vi "Start.vi"(8 "error in (no error)":errorcluster, 10 "Message in":refnum<class "StartMessage.lvclass">, 11 "DAQMH121119OrcaFlash in":refnum<class "DAQOrcaFlash.lvclass">) -> (0 "error out":errorcluster, 3 "DAQMH121119OrcaFlash out":refnum<class "DAQOrcaFlash.lvclass">)   [LabVIEW 2012, in "DAQOrcaFlash.lvclass"]
doc: "This member function is called when the statemachine in the run.vi receives an 'start' command. It relays the message to all observers of the component.\n\nOverride this member function in your derived class if you need additional start functionality (but don't forget to call the parent method)."
uses:
  DAQOrcaFlash.lvclass
  <vilib>/Distrio/Murmex/StartMessage/StartMessage.lvclass
  <vilib>/Distrio/Murmex/Murmex/Murmex.lvclass
  DAQOrcaFlash.lvclass/DAQOrcaFlash.ctl
  imaging_mode.ctl
  trigger_source.ctl
  trigger_mode.ctl
  <vilib>/Distrio/Murmex/ResetMessage/ResetMessage.lvclass
  <vilib>/Distrio/Murmex/Message/Message.lvclass
panel:
  # "This method is called when the START\ntrigger is sent. \n\nOverride this method when your component needs to\nrespond to this trigger. \n\nCall parent for proper implementation"
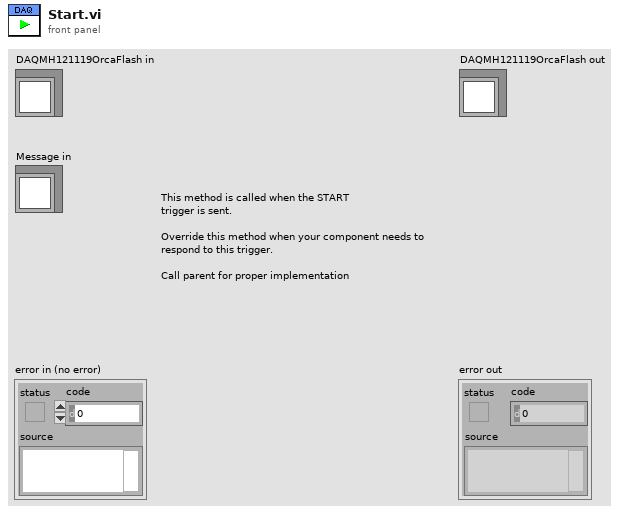
[diagram p1: front panel]
types:
  T1 = typedef "DAQOrcaFlash.lvclass/imaging_mode.ctl" = enum16{"focus mode", "single sweep"}
  T2 = typedef "Murmex.lvlib/StartMessage.lvclass/run mode enum.ctl" = enum16{"infinite", "finite"}
  T3 = typedef "DAQOrcaFlash.lvclass/trigger_mode.ctl" = sgl
  T4 = typedef "DAQOrcaFlash.lvclass/trigger_source.ctl" = sgl
  T5 = typedef "IMAQ Image.ctl" = refnum<image>
  T6 = cluster{"height":u32, "width":u32, "datatype":u32}
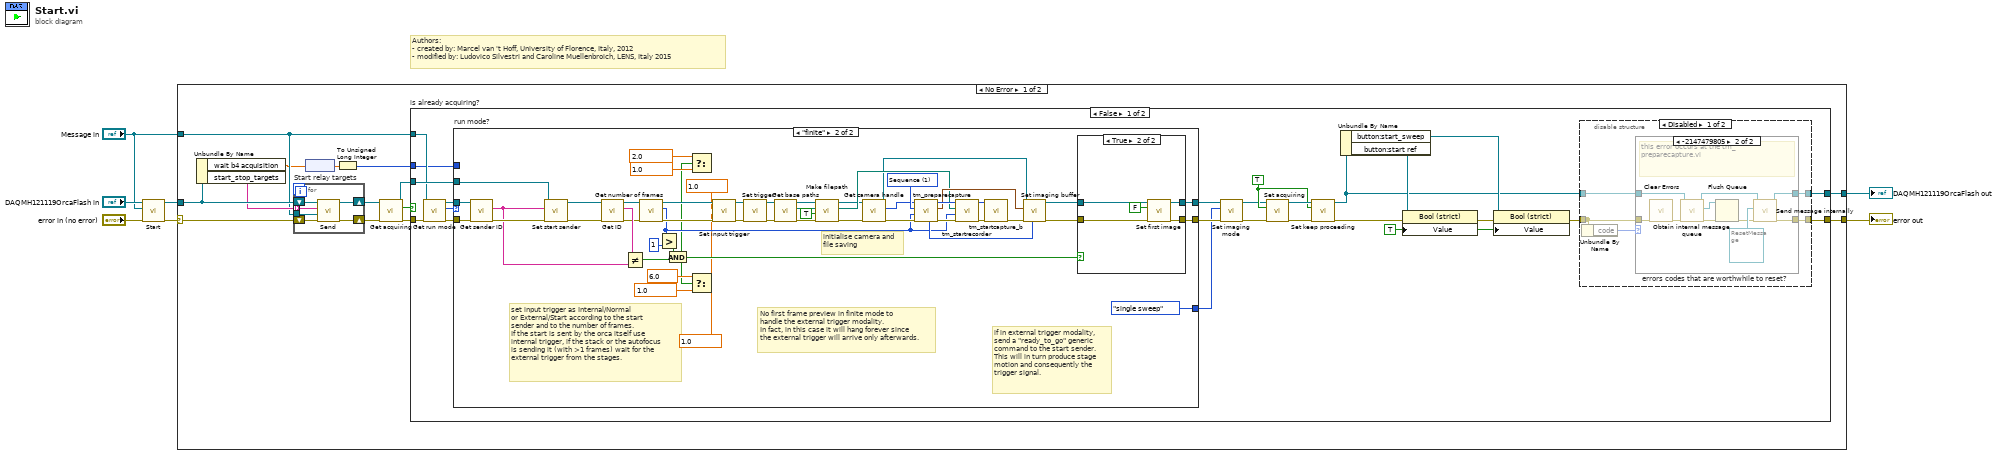
[diagram p0: block diagram]
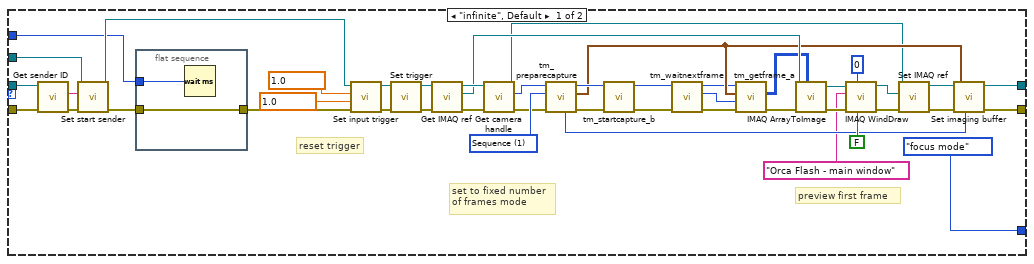
[diagram p4: hidden frame]
diagram:
  # "Authors: \n- created by: Marcel van 't Hoff, University of Florence, Italy, 2012\n- modified by: Ludovico Silvestri and Caroline Muellenbroich, LENS, Italy 2015"
  n1 = call-parent "Start.vi"("error in (no error)"="error in (no error)", "Message in"="Message in", "Murmex in"="DAQMH121119OrcaFlash in") -> ("error out"=w3:errorcluster, "Murmex out"=w4:refnum<class "DAQOrcaFlash.lvclass">)  [unwired: 7 in]
  n2 = case shown="No Error" w3 {
    selector: w3 -> [w14 w178]
    tunnel: [w21 w178] -> w2
    tunnel: [w20 w177] -> w7
    tunnel: w4 -> [w16 w177]
    tunnel: "Message in" -> [w13 _]
    frame No Error {
      n3 = Unbundle By Name(w16) -> ("wait b4 acquisition"=w12:dbl[unit], "start_stop_targets"=w15:string[])
      n4 = for "Start relay targets" {
        shift-right: [w27] -> w9
        shift-left: w14 -> [w26]
        tunnel: w13 -> [w24]
        tunnel: w15 -> [w23] mode=indexing
        shift-right: [w22] -> w10
        shift-left: w16 -> [w25]
        n5 = call <vilib>:"Send.vi"("error in (no error)"=w26, "Message"=w24, "recipient"=w23, "Murmex in"=w25) -> ("error out"=w27:errorcluster, "Murmex out"=w22:refnum<class "DAQOrcaFlash.lvclass">)  [unwired: 6 in]
      }
      n6 = node(w12) -> (w11:dbl)
      n7 = To Unsigned Long Integer(number=w11) -> (unsigned 32bit integer=w8:u32)
      n8 = call "Get acquiring.vi"("error in (no error)"=w9, "DAQMH121119OrcaFlash in"=w10) -> ("error out"=w18:errorcluster, "is acquiring?"=w17:bool, "DAQMH121119OrcaFlash out"=w19:refnum<class "DAQOrcaFlash.lvclass">)  [unwired: 7 in]
      n9 = case "is already acquiring?" shown="False" w17 {
        tunnel: [w38 w176] -> w21
        tunnel: [w36 w175] -> w20
        tunnel: w19 -> [w46 w175]
        tunnel: w18 -> [w42 w176]
        tunnel: w13 -> [w39 _]
        tunnel: w8 -> [w32 _]
        frame False {
          w49 = TRUE ("Value")
          w33 = TRUE ("is acquiring?")
          n10 = call <vilib>:"Get run mode.vi"("error in (no error)"=w42, "StartMessage in"=w39) -> ("error out"=w41:errorcluster, "run mode"=w40:T2, "StartMessage out"=w35:refnum<class "StartMessage.lvclass">)  [unwired: 7 in]
          n11 = case "run mode?" shown="\"finite\"" w40 {
            tunnel: w41 -> [w77 w152]
            tunnel: [w112 w128] -> w51
            tunnel: [w113 w126] -> w45
            tunnel: w46 -> [w75 w124]
            tunnel: [imaging_mode."focus mode" ("imaging mode") imaging_mode."single sweep" ("imaging mode")] -> w44
            tunnel: w35 -> [w76 w151]
            tunnel: w32 -> [w71 _]
            frame "infinite", Default {
              w80 = T3 1.0 items=["Normal"=1.0, "Start"=6.0] ("Trigger mode")
              w81 = T4 1.0 items=["Internal"=1.0, "External"=2.0, "Software"=3.0] ("Trigger source")
              w105 = 1 items=["Snap", "Sequence"] ("Capture mode")
              # "reset trigger"
              # "preview first frame"
              # "set to fixed number\nof frames mode"
              n12 = call <vilib>:"Get sender ID.vi"("error in (no error)"=w77, "Message in"=w76) -> ("error out"=w79:errorcluster, "sender"=w78:string)  [unwired: 7 in, 1 out]
              n13 = call-dynamic "Set start sender.vi"("error in (no error)"=w79, "start sender"=w78, "DAQOrcaFlash in"=w75) -> ("error out"=w72:errorcluster, "DAQOrcaFlash out"=w74:refnum<class "DAQOrcaFlash.lvclass">)  [unwired: 7 in]
              n14 = flat-sequence {
                tunnel: [w117] -> w73
                tunnel: w72 -> [w117]
                tunnel: w71 -> [w116]
                frame #0 {
                  n15 = Wait (ms)(milliseconds to wait=w116) -> ()  [unwired: 1 out]
                }
              }
              n16 = call-dynamic "Set input trigger.vi"("error in (no error)"=w73, "Trigger mode"=w80, "Trigger source"=w81, "DAQOrcaFlash in"=w74) -> ("error out"=w83:errorcluster, "DAQOrcaFlash out"=w84:refnum<class "DAQOrcaFlash.lvclass">)  [unwired: 6 in]
              n17 = call-dynamic "Set trigger.vi"("error in (no error)"=w83, "DAQOrcaFlash in"=w84) -> ("error out"=w82:errorcluster, "DAQOrcaFlash out"=w85:refnum<class "DAQOrcaFlash.lvclass">)  [unwired: 8 in]
              n18 = call "Get IMAQ ref.vi"("error in (no error)"=w82, "DAQMH121119OrcaFlash in"=w85) -> ("error out"=w114:errorcluster, "IMAQ reference"=w99:T5, "DAQMH121119OrcaFlash out"=w115:refnum<class "DAQOrcaFlash.lvclass">)  [unwired: 7 in]
              n19 = call "Get camera handle.vi"("error in (no error)"=w114, "DAQMH121119OrcaFlash in"=w115) -> ("error out"=w88:errorcluster, "cam handle"=w89:u32, "DAQMH121119OrcaFlash out"=w92:refnum<class "DAQOrcaFlash.lvclass">)  [unwired: 7 in]
              n20 = call <userlib>:"tm_preparecapture.vi"("error in (no error)"=w88, "Capture mode"=w105, "Handle in"=w89) -> ("error out"=w106:errorcluster, "Buffer Info"=w97:T6, "Handle out"=w104:u32, "Image type"=w96:u32)  [unwired: 5 in]
              n21 = call <userlib>:"tm_startcapture_b.vi"("error in (no error)"=w106, "Handle in"=w104) -> ("error out"=w102:errorcluster, "Handle out"=w103:u32)  [unwired: 8 in]
              n22 = call <userlib>:"tm_waitnextframe.vi"("error in (no error)"=w102, "Handle in"=w103) -> ("error out"=w87:errorcluster, "Frame Index"=w101:i32, "Handle out"=w86:u32)  [unwired: 6 in, 1 out]
              n23 = call <userlib>:"tm_getframe_a.vi"("error in (no error)"=w87, "Frame Index"=w101, "Buffer Info"=w97, "Handle in"=w86) -> ("error out"=w93:errorcluster, "Data 16"=w95:u16[][])  [unwired: 3 in, 3 out]
              n24 = call "IMAQ ArrayToImage"("Image Pixels (U16)"=w95, "error in (no error)"=w93, "Image"=w99) -> ("error out"=w100:errorcluster, "Image Out"=w98:T5)  [unwired: 7 in]
              n25 = call "IMAQ WindDraw"("Resize to Image Size? (Y)"=FALSE, "Window Number (0...15)"=0, "error in (no error)"=w100, "Title"="Orca Flash - main window", "Image"=w98) -> ("error out"=w108:errorcluster, "Image Out (duplicate)"=w94:T5)  [unwired: 5 in]
              n26 = call "Set IMAQ ref.vi"("error in (no error)"=w108, "IMAQ reference"=w94, "DAQMH121119OrcaFlash in"=w92) -> ("error out"=w109:errorcluster, "DAQMH121119OrcaFlash out"=w110:refnum<class "DAQOrcaFlash.lvclass">)  [unwired: 7 in]
              n27 = call "Set imaging buffer.vi"("Image type"=w96, "error in (no error)"=w109, "Buffer"=w97, "DAQMH121119OrcaFlash in"=w110) -> ("error out"=w112:errorcluster, "DAQMH121119OrcaFlash out"=w113:refnum<class "DAQOrcaFlash.lvclass">)  [unwired: 6 in]
            }
            frame "finite" {
              w118 = T3 1.0 items=["Normal"=1.0, "Start"=6.0] ("Trigger mode")
              w119 = T4 1.0 items=["Internal"=1.0, "External"=2.0, "Software"=3.0] ("Trigger source")
              w142 = T3 1.0 items=["Normal"=1.0, "Start"=6.0] ("Trigger mode")
              w143 = T3 6.0 items=["Normal"=1.0, "Start"=6.0] ("Trigger mode")
              w145 = T4 1.0 items=["Internal"=1.0, "External"=2.0, "Software"=3.0] ("Trigger source")
              w144 = T4 2.0 items=["Internal"=1.0, "External"=2.0, "Software"=3.0] ("Trigger source")
              w165 = 1 items=["Snap", "Sequence"] ("Capture mode")
              # "if in external trigger modality,\nsend a \"ready_to_go\" generic\ncommand to the start sender.\nThis will in turn produce stage\nmotion and consequently the\ntrigger signal."
              # "No first frame preview in finite mode to\nhandle the external trigger modality.\nIn fact, in this case it will hang forever since\nthe external trigger will arrive only afterwards."
              # "set input trigger as Internal/Normal\nor External/Start according to the start\nsender and to the number of frames.\nIf the start is sent by the orca itself use\ninternal trigger, if the stack or the autofocus\nis sending it (with >1 frames) wait for the \nexternal trigger from the stages."
              # "initialise camera and\nfile saving"
              n28 = call <vilib>:"Get sender ID.vi"("error in (no error)"=w152, "Message in"=w151) -> ("error out"=w122:errorcluster, "sender"=w120:string)  [unwired: 7 in, 1 out]
              n29 = call-dynamic "Set start sender.vi"("error in (no error)"=w122, "start sender"=w120, "DAQOrcaFlash in"=w124) -> ("error out"=w121:errorcluster, "DAQOrcaFlash out"=w123:refnum<class "DAQOrcaFlash.lvclass">)  [unwired: 7 in]
              n30 = call <vilib>:"Get ID.vi"("error in (no error)"=w121, "Murmex in"=w123) -> ("error out"=w139:errorcluster, "component id"=w150:string, "Murmex out"=w141:refnum<class "DAQOrcaFlash.lvclass">)  [unwired: 7 in]
              n31 = Not Equal?(x=w150, y=w120) -> (x != y?=w133:bool)
              n32 = call "Get number of frames.vi"("error in (no error)"=w139, "DAQMH121119OrcaFlash in"=w141) -> ("error out"=w138:errorcluster, "no. of frames"=w135:i32, "DAQMH121119OrcaFlash out"=w140:refnum<class "DAQOrcaFlash.lvclass">)  [unwired: 7 in]
              n33 = Greater?(x=w135, y=1) -> (0:w132:bool)
              n34 = And(x=w132, y=w133) -> (x .and. y?=w125:bool)
              n35 = Select(t=w144, s=w125, f=w145) -> ()  [unwired: 1 out]
              n36 = Select(t=w143, s=w125, f=w142) -> ()  [unwired: 1 out]
              n37 = call-dynamic "Set input trigger.vi"("error in (no error)"=w138, "Trigger mode"=w118, "Trigger source"=w119, "DAQOrcaFlash in"=w140) -> ("error out"=w146:errorcluster, "DAQOrcaFlash out"=w147:refnum<class "DAQOrcaFlash.lvclass">)  [unwired: 6 in]
              n38 = call-dynamic "Set trigger.vi"("error in (no error)"=w146, "DAQOrcaFlash in"=w147) -> ("error out"=w149:errorcluster, "DAQOrcaFlash out"=w148:refnum<class "DAQOrcaFlash.lvclass">)  [unwired: 8 in]
              n39 = call-dynamic "Get base paths.vi"("error in (no error)"=w149, "DAQOrcaFlash in"=w148) -> ("error out"=w161:errorcluster, "filepath"=w159:path, "DAQOrcaFlash out"=w160:refnum<class "DAQOrcaFlash.lvclass">)  [unwired: 6 in, 1 out]
              n40 = call "Make filepath.vi"("error in (no error)"=w161, "is cxd file path?"=TRUE, "base path"=w159, "DAQOrcaFlash in"=w160) -> ("error out"=w136:errorcluster, "filepath out"=w158:path, "DAQOrcaFlash out"=w137:refnum<class "DAQOrcaFlash.lvclass">)  [unwired: 5 in]
              n41 = call "Get camera handle.vi"("error in (no error)"=w136, "DAQMH121119OrcaFlash in"=w137) -> ("error out"=w154:errorcluster, "cam handle"=w155:u32, "DAQMH121119OrcaFlash out"=w130:refnum<class "DAQOrcaFlash.lvclass">)  [unwired: 7 in]
              n42 = call <userlib>:"tm_preparecapture.vi"("error in (no error)"=w154, "Frames"=w135, "Capture mode"=w165, "Handle in"=w155) -> ("error out"=w166:errorcluster, "Buffer Info"=w162:T6, "Handle out"=w167:u32, "Image type"=w163:u32)  [unwired: 4 in]
              n43 = call <userlib>:"tm_startrecorder.vi"("error in (no error)"=w166, "frames"=w135, "File"=w158, "Handle in"=w167) -> ("error out"=w156:errorcluster, "Handle out"=w157:u32)  [unwired: 6 in]
              n44 = call <userlib>:"tm_startcapture_b.vi"("error in (no error)"=w156, "Handle in"=w157) -> ("error out"=w131:errorcluster)  [unwired: 8 in, 1 out]
              n45 = call "Set imaging buffer.vi"("Image type"=w163, "error in (no error)"=w131, "Buffer"=w162, "DAQMH121119OrcaFlash in"=w130) -> ("error out"=w129:errorcluster, "DAQMH121119OrcaFlash out"=w127:refnum<class "DAQOrcaFlash.lvclass">)  [unwired: 6 in]
              n46 = case shown="True" w125 {
                tunnel: w129 -> [w168 w171]
                tunnel: [w168 w174] -> w128
                tunnel: w127 -> [w169 w170]
                tunnel: [w169 w173] -> w126
                frame False {
                }
                frame True {
                  n47 = call-dynamic "Set first image.vi"("error in (no error)"=w171, "first image acquired?"=FALSE, "DAQOrcaFlash in"=w170) -> ("error out"=w174:errorcluster, "DAQOrcaFlash out"=w173:refnum<class "DAQOrcaFlash.lvclass">)  [unwired: 7 in]
                }
              }
            }
          }
          n48 = call "Set imaging mode.vi"("error in (no error)"=w51, "imaging mode"=w44, "DAQMH121119OrcaFlash in"=w45) -> ("error out"=w30:errorcluster, "DAQMH121119OrcaFlash out"=w31:refnum<class "DAQOrcaFlash.lvclass">)  [unwired: 7 in]
          n49 = call "Set acquiring.vi"("error in (no error)"=w30, "is acquiring?"=w33, "DAQMH121119OrcaFlash in"=w31) -> ("error out"=w43:errorcluster, "DAQMH121119OrcaFlash out"=w34:refnum<class "DAQOrcaFlash.lvclass">)  [unwired: 7 in]
          n50 = call-dynamic "Set keep proceeding.vi"("error in (no error)"=w43, "keep proceeding?"=w33, "DAQOrcaFlash in"=w34) -> ("error out"=w28:errorcluster, "DAQOrcaFlash out"=w29:refnum<class "DAQOrcaFlash.lvclass">)  [unwired: 7 in]
          n51 = Unbundle By Name(w29) -> ("button:start_sweep"=w47:refnum<vi>, "button:start ref"=w50:refnum<vi>)
          n52 = property class="Bool (strict)"(reference=w50, error in=w28, "Value"=w49) -> (error out=w48:errorcluster)  [unwired: 1 out]
          n53 = property class="Bool (strict)"(reference=w47, error in=w48, "Value"=w49) -> (error out=w37:errorcluster)  [unwired: 1 out]
          n54 = disable-structure shown="Disabled" {
            disable-tunnel: [w56 w69] -> w38
            disable-tunnel: w37 -> [w55 w69]
            disable-tunnel: w29 -> [w54 w70]
            disable-tunnel: [w53 w70] -> w36
            frame Disabled {
              n55 = Unbundle By Name(w55) -> ("code"=w52:i32)
              n56 = case "errors codes that are worthwhile to reset?" shown="-2147479805" w52 {
                tunnel: [w58 w67] -> w56
                tunnel: w55 -> [w58 w68]
                tunnel: w54 -> [w57 w64]
                tunnel: [w57 w66] -> w53
                frame Default {
                }
                frame -2147479805 {
                  # "this error occurs at the tm_preparecapture.vi"
                  n57 = call <vilib>:"Clear Errors.vi"("error in (no error)"=w68) -> ("error out"=w63:errorcluster)  [unwired: 6 in]
                  n58 = call <vilib>:"Obtain internal message queue.vi"("error in (no error)"=w63, "Murmex in"=w64) -> ("error out"=w60:errorcluster, "internal message queue"=w61:refnum<queue>, "Murmex out"=w62:refnum<class "DAQOrcaFlash.lvclass">)  [unwired: 7 in]
                  n59 = Flush Queue(queue=w61, error in (no error)=w60) -> (error out=w59:errorcluster)  [unwired: 2 out]
                  n60 = call <vilib>:"Send message internally.vi"("error in (no error)"=w59, "Message"=refnum<class "ResetMessage.lvclass"> refnum ("Message in"), "Murmex in"=w62) -> ("error out"=w67:errorcluster, "Murmex out"=w66:refnum<class "DAQOrcaFlash.lvclass">)  [unwired: 7 in]
                }
              }
            }
            frame Enabled {
            }
          }
        }
        frame True {
          # "Skip double start trigger events"
        }
      }
    }
    frame Error {
    }
  }
  "DAQMH121119OrcaFlash out" <- w7
  "error out" <- w2
